vi "Draw.vi"(8 "error in (no error)":errorcluster, 9 "Text":string, 10 "Bars":T1[][](array[typedef]), 11 "2D Barcode in":refnum<class "BarCode.lvclass">) -> (0 "error out":errorcluster, 2 "new picture":picture, 3 "2D Barcode out":refnum<class "BarCode.lvclass">)   [LabVIEW 2013, in "BarCodes.lvlib" / "BarCode.lvclass"]
uses:
  BarCode.lvclass
  Bar.ctl
  Read Scale.vi
  Read Light Color.vi
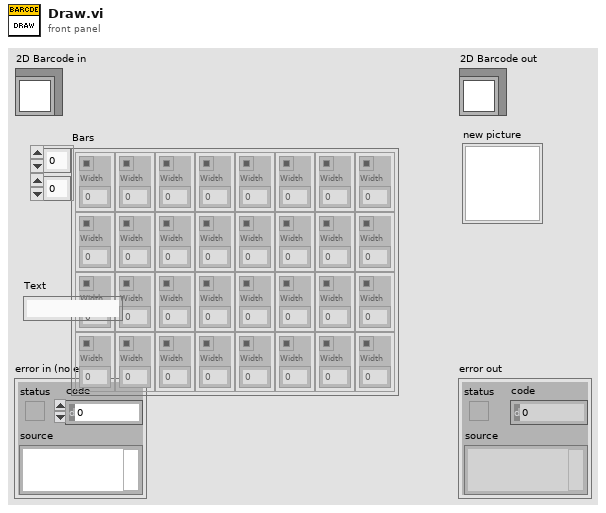
[diagram p1: front panel]
types:
  T1 = typedef "BarCodes.lvlib/BarCode.lvclass/Bar.ctl" = cluster{"Color":u32, "Width":u8}
  T2 = cluster{"Width":i16, "Style":enum32{"Solid", "Dash", "Dot", "DashDot", "DashDotDot"}}
  T3 = cluster{"left":i16, "top":i16, "right":i16, "bottom":i16}
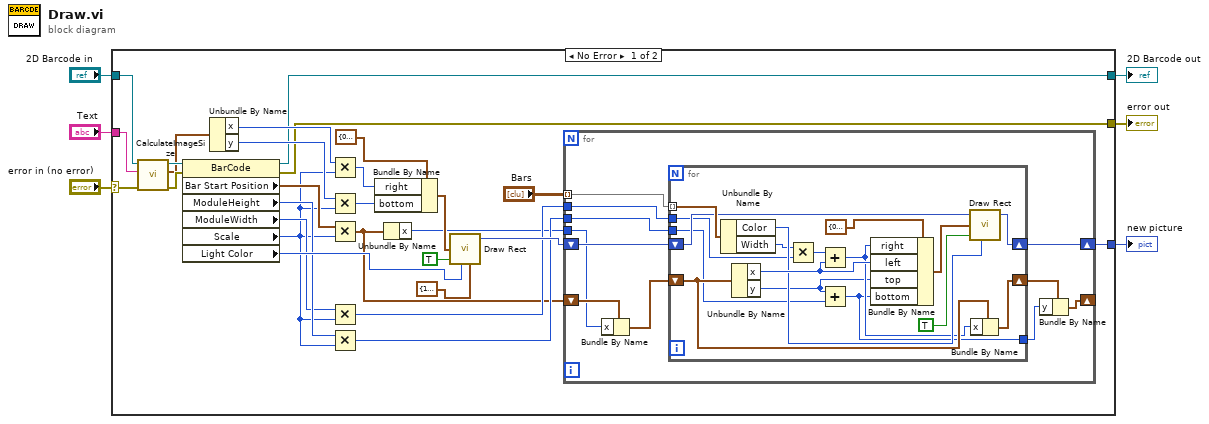
[diagram p0: block diagram]
diagram:
  n1 = case shown="No Error" "error in (no error)" {
    selector: "error in (no error)" -> [w32 w64]
    tunnel: "2D Barcode in" -> [w34 w63]
    tunnel: "Text" -> [w33 _]
    tunnel: [w9 w64] -> w3
    tunnel: [w8 w63] -> w2
    tunnel: [w7 _] -> w1
    frame No Error {
      n2 = call-dynamic "CalculateImageSize.vi"("error in (no error)"=w32, "String"=w33, "BarCode in"=w34) -> ("error out"=w30:errorcluster, "Size"=w29:cluster{"x":i16, "y":i16}, "BarCode out"=w31:refnum<class "BarCode.lvclass">)  [unwired: 6 in]
      n3 = property class="BarCode"(reference=w31, error in=w30) -> (reference out=w8:refnum<class "BarCode.lvclass">, error out=w9:errorcluster, "Bar Start Position"=w19:cluster{"x":i16, "y":i16}, "ModuleHeight"=w16:u8, "ModuleWidth"=w15:u8, "Scale"=w12:u8, "Light Color"=w21:u32)
      n4 = Unbundle By Name(w29) -> ("x"=w24:i16, "y"=w25:i16)
      n5 = Multiply(x=w24, y=w12) -> (x*y=w28:i16)
      n6 = Multiply(x=w25, y=w12) -> (x*y=w27:i16)
      n7 = Multiply(x=w19, y=w12) -> (x*y=w11:cluster{"x":i16, "y":i16})
      n8 = Multiply(x=w15, y=w12) -> (x*y=w13:u8)
      n9 = Multiply(x=w16, y=w12) -> (x*y=w14:u8)
      n10 = Bundle By Name(cluster=T3 {"left"=0, "top"=0, "right"=0, "bottom"=0} ("rect"), "right"=w28, "bottom"=w27) -> (w23:T3)
      n11 = Unbundle By Name(w11) -> ("x"=w10:i16)
      n12 = call <vilib>:"Draw Rect.vi"("rect"=w23, "fill?(F)"=TRUE, "color(black)"=w21, "pen"=T2 {"Width"=1, "Style"=enum."Solid"}) -> ("new picture"=w18:picture)  [unwired: 5 in]
      n13 = for {
        shift-right: [w35] -> w7
        shift-left: w18 -> [w44]
        tunnel: "Bars" -> [w45] mode=indexing
        tunnel: w14 -> [w39]
        tunnel: w13 -> [w43]
        shift-right: [w38] -> _
        shift-left: w11 -> [w42]
        tunnel: w10 -> [w41]
        n14 = Bundle By Name(cluster=w42, "x"=w41) -> (w40:cluster{"x":i16, "y":i16})
        n15 = for {
          tunnel: w45 -> [w62] mode=indexing
          shift-right: [w56] -> w35
          shift-left: w44 -> [w57]
          tunnel: w43 -> [w47]
          shift-right: [w51] -> w37
          shift-left: w40 -> [w53]
          tunnel: w39 -> [w46]
          tunnel: [w50] -> w36
          n16 = Unbundle By Name(w62) -> ("Color"=w54:u32, "Width"=w49:u8)
          n17 = Unbundle By Name(w53) -> ("x"=w59:i16, "y"=w48:i16)
          n18 = Multiply(x=w49, y=w47) -> (x*y=w60:u8)
          n19 = Add(x=w60, y=w59) -> (x+y=w52:i16)
          n20 = Add(x=w48, y=w46) -> (x+y=w50:i16)
          n21 = Bundle By Name(cluster=T3 {"left"=0, "top"=0, "right"=0, "bottom"=0} ("rect"), "right"=w52, "left"=w59, "top"=w48, "bottom"=w50) -> (w58:T3)
          n22 = call <vilib>:"Draw Rect.vi"("picture"=w57, "rect"=w58, "fill?(F)"=TRUE, "color(black)"=w54) -> ("new picture"=w56:picture)  [unwired: 5 in]
          n23 = Bundle By Name(cluster=w53, "x"=w52) -> (w51:cluster{"x":i16, "y":i16})
        }
        n24 = Bundle By Name(cluster=w37, "y"=w36) -> (w38:cluster{"x":i16, "y":i16})
      }
    }
    frame Error {
    }
  }
  "error out" <- w3
  "2D Barcode out" <- w2
  "new picture" <- w1
